vi "IEEE754_lesen.vi"(8 "lo":u16[](array[numeric]), 11 "hi":u16[](array[numeric])) -> (3 "Werte":sgl[](array[numeric]) format="%#.3f")   [LabVIEW 2020, in "ABB-EL3000.lvlib" / "Allgemeine VI.lvlib"]
uses:
  Allgemeine VI.lvlib
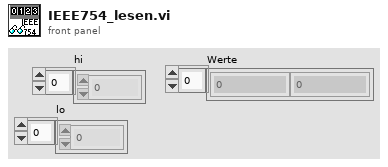
[diagram p1: front panel]
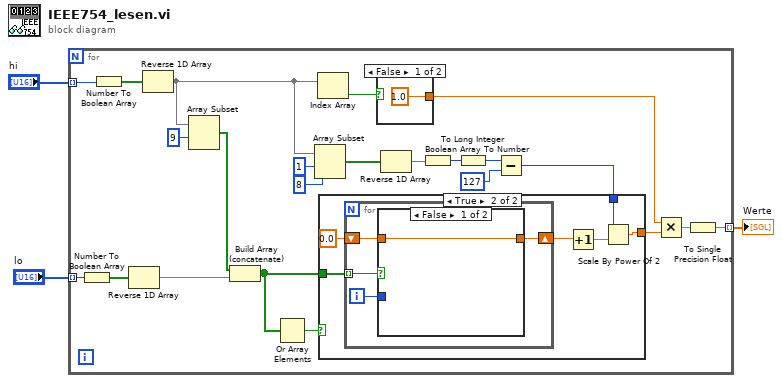
[diagram p0: block diagram]
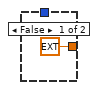
[diagram p2: hidden frame]
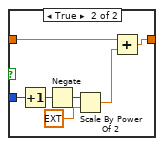
[diagram p3: hidden frame]
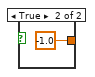
[diagram p4: hidden frame]
diagram:
  n1 = for {
    tunnel: [w6] -> w3 mode=indexing
    tunnel: "lo" -> [w9] mode=indexing
    tunnel: "hi" -> [w8] mode=indexing
    n2 = Number To Boolean Array(number=w9) -> (Boolean array=w25:bool[])
    n3 = Number To Boolean Array(number=w8) -> (Boolean array=w26:bool[])
    n4 = Reverse 1D Array(array=w25) -> (reversed array=w14:bool[])
    n5 = Reverse 1D Array(array=w26) -> (reversed array=w16:bool[])
    n6 = Array Subset(array=w16, index=9 ("Index")) -> (w13:bool[])  [unwired: 1 in]
    n7 = Build Array (concatenate)(w13, w14) -> (w5:bool[])
    n8 = Or Array Elements(Boolean array=w5) -> (logical OR=w4:bool)
    n9 = Array Subset(array=w16, index=1 ("Index"), length=8 ("Länge")) -> (w21:bool[])
    n10 = Index Array(array=w16) -> (element=w24:bool)  [unwired: 1 in]
    n11 = case shown="False" w24 {
      tunnel: [1.0 -1.0] -> w11
      frame False {
      }
      frame True {
      }
    }
    n12 = Reverse 1D Array(array=w21) -> (reversed array=w20:bool[])
    n13 = Boolean Array To Number(Boolean array=w20) -> (number=w19:u32)
    n14 = To Long Integer(number=w19) -> (32bit integer=w18:i32)
    n15 = Subtract(x=w18, y=127) -> (x-y=w12:i32)
    n16 = case shown="True" w4 {
      tunnel: w5 -> [_ w33]
      tunnel: w12 -> [_ w29]
      tunnel: [ext 0.0 w28] -> w10
      frame False {
      }
      frame True {
        n17 = for {
          tunnel: w33 -> [w37] mode=indexing
          shift-right: [w34] -> w31
          shift-left: 0.0 -> [w35]
          i -> [w36]
          n18 = case shown="False" w37 {
            tunnel: w36 -> [_ w45]
            tunnel: w35 -> [w38 w40]
            tunnel: [w38 w41] -> w34
            frame False {
            }
            frame True {
              n19 = Increment(x=w45) -> (x+1=w44:i32)
              n20 = Negate(x=w44) -> (-x=w43:i32)
              n21 = Scale By Power Of 2(n=w43, x=ext 1.0) -> (x*2^n=w39:ext)
              n22 = Add(x=w40, y=w39) -> (x+y=w41:ext)
            }
          }
        }
        n23 = Increment(x=w31) -> (x+1=w30:ext)
        n24 = Scale By Power Of 2(n=w29, x=w30) -> (x*2^n=w28:ext)
      }
    }
    n25 = Multiply(x=w11, y=w10) -> (x*y=w7:ext)
    n26 = To Single Precision Float(number=w7) -> (single precision float=w6:sgl)
  }
  "Werte" <- w3
